vi "ReadAll.vi"(4 "TypeMap in":refnum<class "TypeMap.lvclass">, 5 "Select *":bool=TRUE, 6 "commandTimeout":i32, 7 "Where":string, 8 "error in (no error)":errorcluster, 9 "Limit":i64, 10 "object in":refnum<class>, 11 "SqlMapper in":refnum<class "SqlMapper.lvclass">) -> (0 "error out":errorcluster, 2 "Query Result out":refnum<class "Query Result.lvclass">, 3 "SqlMapper out":refnum<class "SqlMapper.lvclass">)   [LabVIEW 2020, in "ORM.lvlib" / "TypeMap.lvclass"]
uses:
  TypeMap.lvclass
  SqlMapper/SqlMapper.lvclass
  Query Result/Query Result.lvclass
  Read KeyProperties.vi
  Read Table Name.vi
  DynamicParameters/DynamicParameters.lvclass
  TypeMap.lvclass/TypeMap.ctl
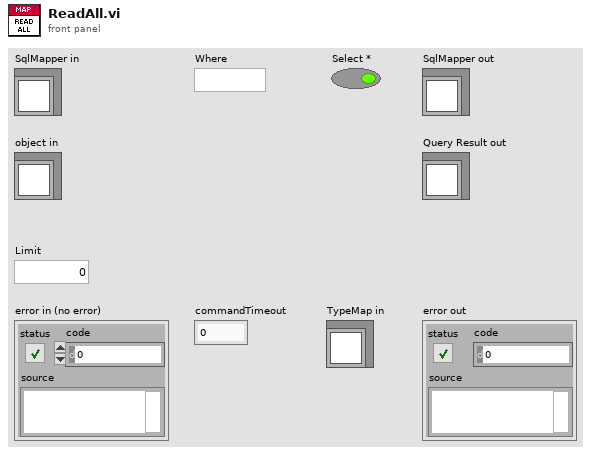
[diagram p1: front panel]
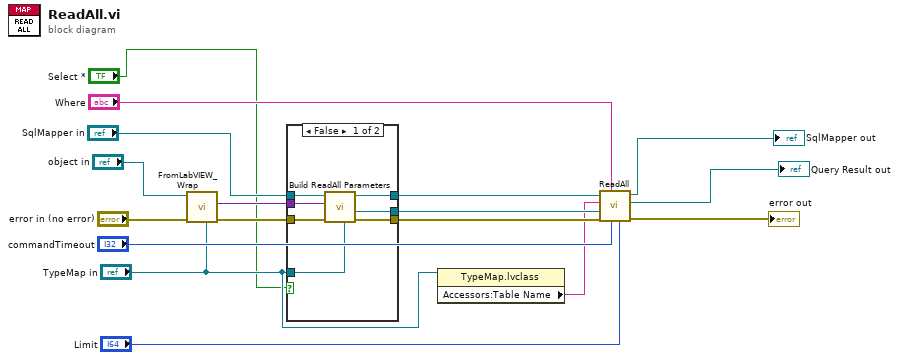
[diagram p0: block diagram]
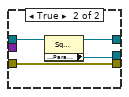
[diagram p2: hidden frame]
diagram:
  n1 = call "FromLabVIEW_Wrap.vi"("TypeMap in"="TypeMap in", "error in (no error)"="error in (no error)", "object in"="object in") -> ("error out"=w14:errorcluster, "DbRow"=w15:variant)  [unwired: 7 in]
  n2 = case shown="False" "Select *" {
    tunnel: "SqlMapper in" -> [w24 w28]
    tunnel: w15 -> [w23 _]
    tunnel: w14 -> [w22 w27]
    tunnel: [w21 w27] -> w11
    tunnel: [w20 w26] -> w10
    tunnel: [w19 w25] -> w8
    tunnel: "TypeMap in" -> [w18 _]
    frame False {
      n3 = call-dynamic "Build ReadAll Parameters.vi"("TypeMap in"=w18, "error in (no error)"=w22, "object"=w23, "SqlMapper in"=w24) -> ("error out"=w21:errorcluster, "DynamicParameters out"=w19:refnum<class "DynamicParameters.lvclass">, "SqlMapper out"=w20:refnum<class "SqlMapper.lvclass">)  [unwired: 5 in]
    }
    frame True {
      n4 = property class="SqlMapper.lvclass"(reference=w28) -> (reference out=w26:refnum<class "SqlMapper.lvclass">, "Accessors:Parameter"=w25:refnum<class "DynamicParameters.lvclass">)  [unwired: 1 in, 1 out]
    }
  }
  n5 = property class="TypeMap.lvclass"(reference="TypeMap in") -> ("Accessors:Table Name"=w6:string)  [unwired: 1 in, 2 out]
  n6 = call "ReadAll.vi"("Limit"="Limit", "commandTimeout"="commandTimeout", "Where"="Where", "error in (no error)"=w11, "DynamicParameters"=w8, "TableName"=w6, "SqlMapper in"=w10) -> ("error out"=→"error out":errorcluster, "Query Result out"=→"Query Result out":refnum<class "Query Result.lvclass">, "SqlMapper out"=→"SqlMapper out":refnum<class "SqlMapper.lvclass">)  [unwired: 2 in]
